vi "Day 12-Check if Allowed to go through.vi"(9 "Path in":string[](array[string]), 10 "Cave":string, 11 "Conditions":enum32{"Part 1", "Part 2"}(radio)) -> (3 "Allowed?":bool)   [LabVIEW 2021]
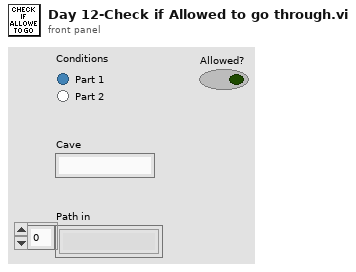
[diagram p1: front panel]
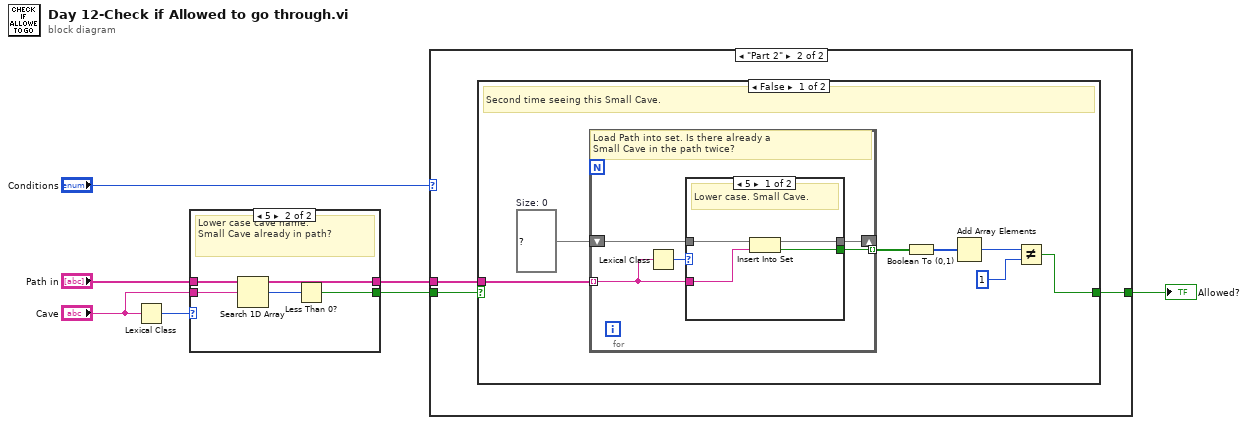
[diagram p0: block diagram]
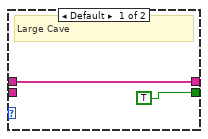
[diagram p2: hidden frame]
diagram:
  n1 = Lexical Class(1:"Cave") -> (0:w4:i16)
  n2 = case shown="5" w4 {
    tunnel: "Path in" -> [w9 w10]
    tunnel: [TRUE w12] -> w2
    tunnel: "Cave" -> [_ w11]
    tunnel: [w9 w10] -> w3
    frame Default {
      # "Large Cave"
    }
    frame 5 {
      # "Lower case cave name.  \nSmall Cave already in path?"
      n3 = Search 1D Array(1D array=w10, element=w11) -> (index of element=w13:i32)  [unwired: 1 in]
      n4 = Less Than 0?(x=w13) -> (x < 0?=w12:bool)
    }
  }
  n5 = case shown="\"Part 2\"" "Conditions" {
    tunnel: [w14 w15] -> w7
    tunnel: w3 -> [_ w17]
    tunnel: w2 -> [w14 w16]
    frame "Part 1" {
    }
    frame "Part 2" {
      n6 = case shown="False" w16 {
        selector: w16 -> [_ w35]
        tunnel: w17 -> [w23 _]
        tunnel: [w18 w35] -> w15
        frame False {
          w24 = set{string} {}  # Size: 0
          # "Second time seeing this Small Cave."
          n7 = for {
            tunnel: w23 -> [w27] mode=indexing
            shift-right: [w28] -> _
            shift-left: w24 -> [w26]
            tunnel: [w25] -> w21 mode=indexing
            # "Load Path into set. Is there already a \nSmall Cave in the path twice?"
            n8 = Lexical Class(1:w27) -> (0:w29:i16)
            n9 = case shown="5" w29 {
              tunnel: [w33 w34] -> w28
              tunnel: w27 -> [w32 _]
              tunnel: w26 -> [w31 w34]
              tunnel: [w30 _] -> w25
              frame 5 {
                # "Lower case. Small Cave."
                n10 = Insert Into Set(10:w32, 11:w31) -> (2:w30:bool, 3:w33:set{string})
              }
              frame Default {
              }
            }
          }
          n11 = Boolean To (0,1)(Boolean=w21) -> (0, 1=w22:i16[])
          n12 = Add Array Elements(numeric array=w22) -> (sum=w20:i16)
          n13 = Not Equal?(x=w20, y=i16 1) -> (x != y?=w18:bool)
        }
        frame True {
          # "Large Cave OR first time seeing this Small Cave."
        }
      }
    }
  }
  "Allowed?" <- w7
